vi "Process-Event.vi"(8 "error in":errorcluster, 11 "DAQmx":refnum<class "DAQmx.lvclass">) -> (0 "error out":errorcluster, 3 "DAQmx out":refnum<class "DAQmx.lvclass">)   [LabVIEW 2019, in "DAQmx.lvclass"]
uses:
  DAQmx.lvclass
  C:/Program Files (x86)/National Instruments/LabVIEW 2019/vi.lib/JKI/JKI SMO/SMO/SMO.lvclass
  typedefs/DAQmx.States--enum.ctl
  typedefs/DAQmx.Status--enum.ctl
  <vilib>/JKI/JKI SMO/SMO/SMO.lvclass/SMO.ctl
  DAQmx.lvclass/DAQmx.ctl
  <vilib>/JKI/JKI SMO/SMO/Private/ReftoDVR--SMO.vi
  <vilib>/JKI/JKI SMO/SMO/Protected/Register Process.vi
  <vilib>/JKI/JKI SMO/SMO/SMO.lvclass
panel:
  out "Current State":string
  out "Status":T1
  out "State":T2
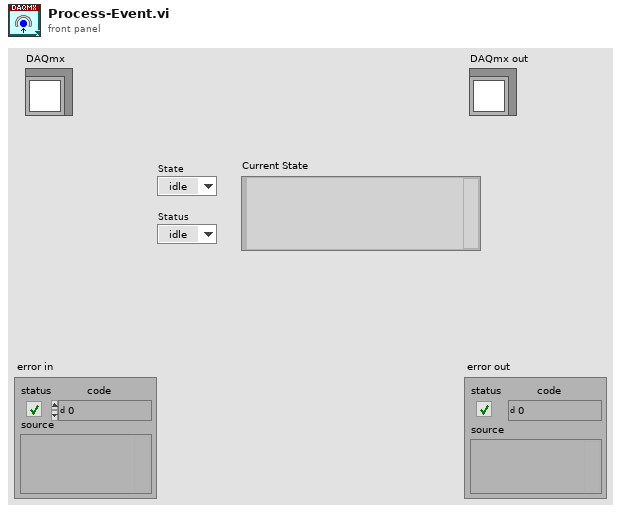
[diagram p1: front panel]
types:
  T1 = typedef "DAQmx.lvclass/DAQmx.Status--enum.ctl" = enum16{"idle", "calibrating", "configuring", "creating", "created", "starting", "started", "stopping", "stopped", "clearing"}
  T2 = typedef "DAQmx.lvclass/DAQmx.States--enum.ctl" = enum16{"idle", "start", "stop", "calibrate", "auto", "exit"}
  T3 = enum32{"Invalid", "Standard", "Closed", "Hidden", "Minimized", "Maximized"}
  T4 = typedef "SMO.lvclass/Protected Events.ctl" = cluster{"StopProcesses":refnum<user-event>, "AbortProcesses":refnum<user-event>, "Config Changed":refnum<user-event>, "Dependency":refnum<user-event>}
  T5 = typedef "DAQmx.lvclass/PrivateEvents--Cluster.ctl" = cluster{"State":refnum<user-event>, "AOconfig":refnum<user-event>, "AIconfig":refnum<user-event>, "Timing":refnum<user-event>}
  T6 = typedef "DAQmx.lvclass/DAQ.Config.AO--Cluster--Array.ctl" = T7[]
  T7 = typedef "DAQmx.lvclass/DAQ.Config.AO--Cluster.ctl" = cluster{"Channels":tag, "Range":T8, "output terminal configuration":i32, "Type":T9}
  T8 = typedef "DAQmx.lvclass/DAQ.Config.AO.Range--enum.ctl" = enum16{"±0.1", "±1.0", "±10.0", ""}
  T9 = typedef "DAQmx.lvclass/DAQ.Config.Device Type--enum.ctl" = enum16{"None", "USB-4431", "PXI-446x"}
  T10 = typedef "DAQmx.lvclass/DAQ.Config.AI--Cluster--Array.ctl" = T11[]
  T11 = typedef "DAQmx.lvclass/DAQ.Config.AI--Cluster.ctl" = cluster{"Channels":tag, "Coupling":T12, "Range":T13, "input terminal configuration":i32, "Type":T9}
  T12 = typedef "DAQmx.lvclass/DAQ.Config.AI.Coupling--enum.ctl" = u16
  T13 = typedef "DAQmx.lvclass/DAQ.Config.AI.Range--enum.ctl" = enum16{"±0.316", "±1.00", "±3.16", "±10.0", "±31.6", "±42.4", ""}
  T14 = typedef "DAQmx.lvclass/DAQ.Config.Timing.Sampling--Cluster.ctl" = cluster{"Fs":dbl, "#s":i32}
  T15 = typedef "DAQmx.lvclass/DeviceInfo--Cluster.ctl" = cluster{"DeviceName":string, "DevIsSimulated":bool, "DeviceSerialNumber":u32, "ProductType":string, "ProductCategory":i32, "ProductNumber":u32, "ChassisNumber":u32, "SlotNumber":u32, "ChassisName":string, "ChassisSerialNumber":u32}
  T16 = typedef "DAQmx.lvclass/DAQ.Calibration--Cluster.ctl" = cluster{"Active Device":string, "SelfCal.LastDate/Time":dbl, "SelfCal.LastTemp":dbl, "DevTemp":dbl, "calibration due?":bool}
  T17 = typedef "DAQmx.lvclass/DAQ.Calibration--Cluster--Array.ctl" = T16[]
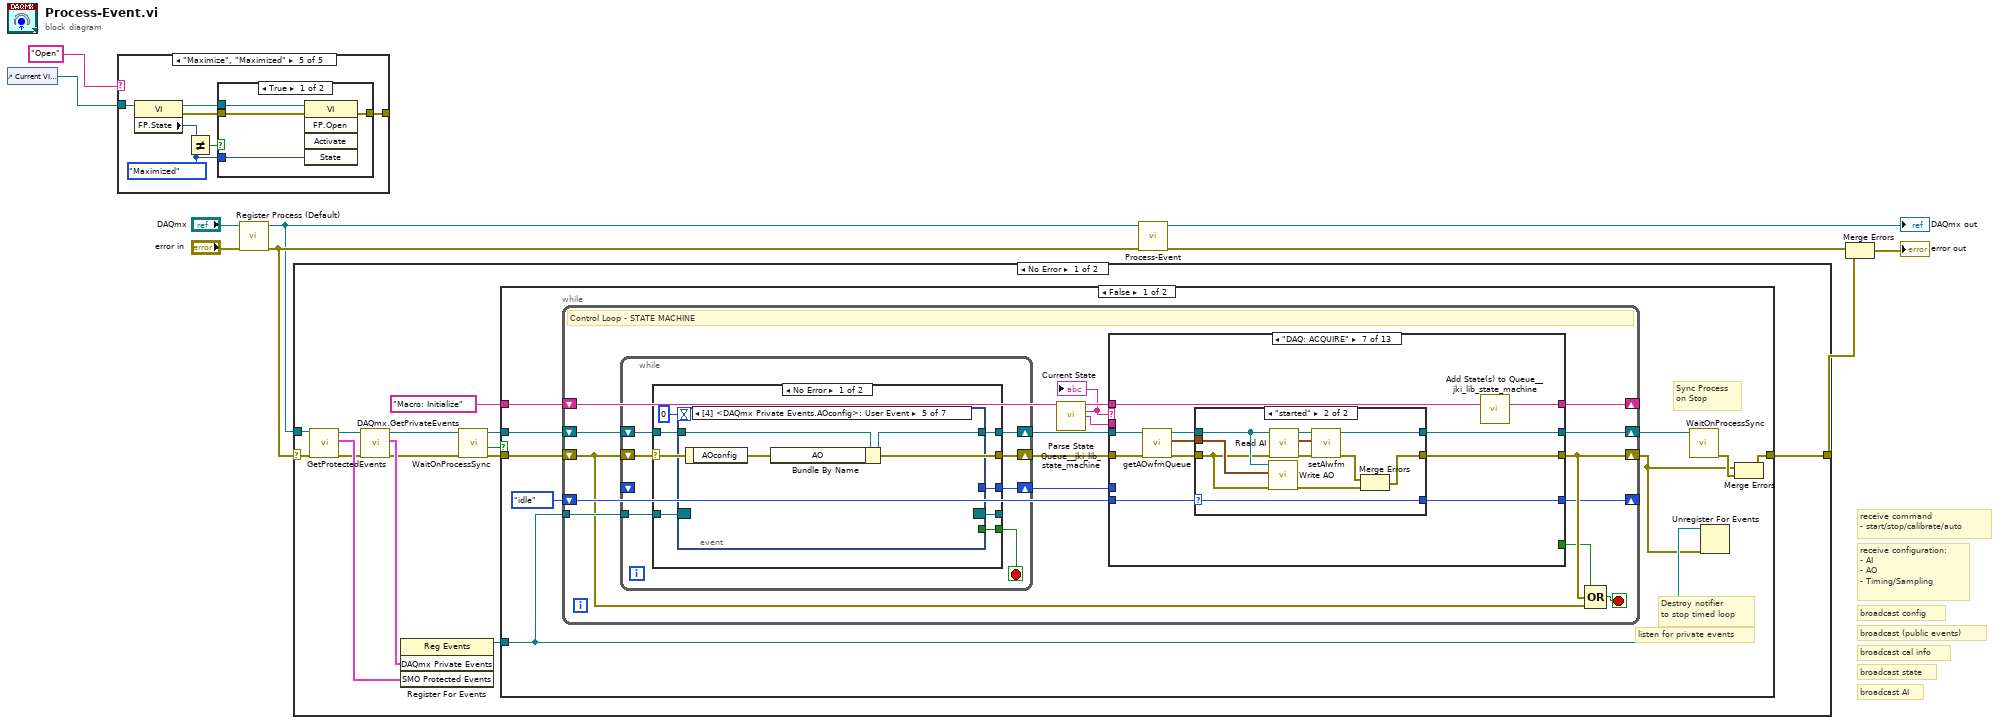
[diagram p0: block diagram]
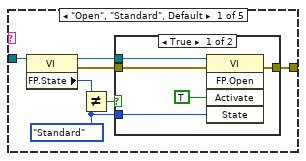
[diagram p2: hidden frame]
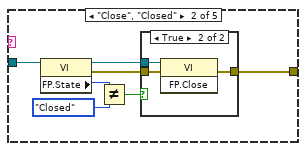
[diagram p4: hidden frame]
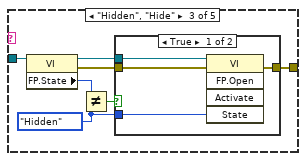
[diagram p6: hidden frame]
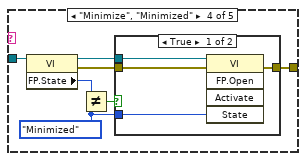
[diagram p8: hidden frame]
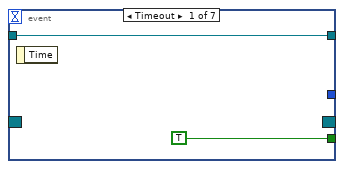
[diagram p11: hidden frame]
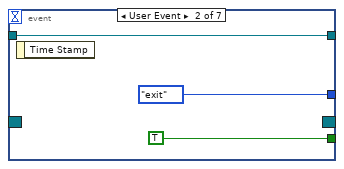
[diagram p12: hidden frame]
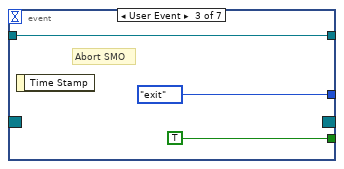
[diagram p13: hidden frame]
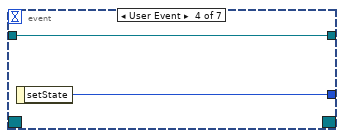
[diagram p14: hidden frame]
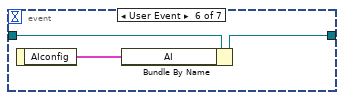
[diagram p15: hidden frame]
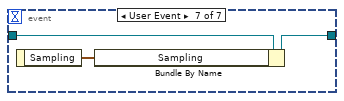
[diagram p16: hidden frame]
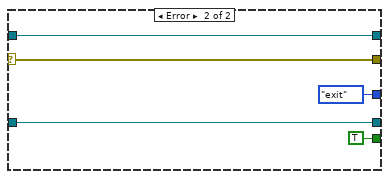
[diagram p17: hidden frame]
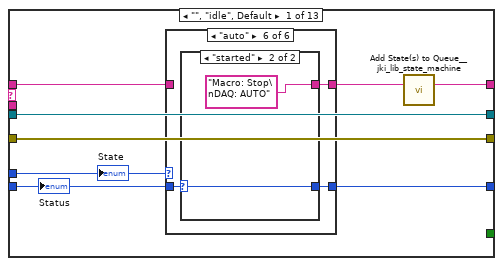
[diagram p18: hidden frame]
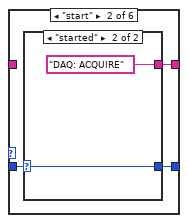
[diagram p20: hidden frame]
diagram:
  # "broadcast (public events)"
  # "receive configuration:\n- AI\n- AO\n- Timing/Sampling"
  # "receive command\n- start/stop/calibrate/auto"
  # "broadcast AI"
  # "broadcast state"
  # "broadcast cal info"
  # "broadcast config"
  n1 = control-ref of="Current VI Reference"() -> (w2:refnum<vi>)
  n2 = case shown="\"Maximize\", \"Maximized\"" "Open" {
    tunnel: [w17 w30 w41 w53 w65] -> _
    tunnel: w2 -> [w16 w28 w40 w52 w64]
    frame "Open", "Standard", Default {
      w11 = T3."Standard" ("State")
      n3 = property class="VI"(reference=w16) -> (reference out=w14:refnum<vi>, error out=w15:errorcluster, "FP.State"=w13:T3)  [unwired: 1 in]
      n4 = Not Equal?(x=w13, y=w11) -> (x != y?=w12:bool)
      n5 = case shown="True" w12 {
        tunnel: [w21 w23] -> w17
        tunnel: w15 -> [w20 w23]
        tunnel: w14 -> [w19 _]
        tunnel: w11 -> [w18 _]
        frame True {
          n6 = invoke class="VI" method="FP.Open"(reference=w19, error in=w20, "Activate"=TRUE, "State"=w18) -> (error out=w21:errorcluster)  [unwired: 1 in, 4 out]
        }
        frame False {
        }
      }
    }
    frame "Close", "Closed" {
      n7 = property class="VI"(reference=w28) -> (reference out=w27:refnum<vi>, error out=w29:errorcluster, "FP.State"=w25:T3)  [unwired: 1 in]
      n8 = Not Equal?(x=w25, y=T3."Closed" ("Front Panel Window:State")) -> (x != y?=w24:bool)
      n9 = case shown="True" w24 {
        tunnel: [w31 w34] -> w30
        tunnel: w29 -> [w31 w33]
        tunnel: w27 -> [_ w32]
        frame False {
        }
        frame True {
          n10 = invoke class="VI" method="FP.Close"(reference=w32, error in=w33) -> (error out=w34:errorcluster)  [unwired: 1 in, 2 out]
        }
      }
    }
    frame "Hidden", "Hide" {
      w35 = T3."Hidden" ("State")
      n11 = property class="VI"(reference=w40) -> (reference out=w38:refnum<vi>, error out=w39:errorcluster, "FP.State"=w37:T3)  [unwired: 1 in]
      n12 = Not Equal?(x=w37, y=w35) -> (x != y?=w36:bool)
      n13 = case shown="True" w36 {
        tunnel: [w45 w46] -> w41
        tunnel: w39 -> [w44 w46]
        tunnel: w38 -> [w43 _]
        tunnel: w35 -> [w42 _]
        frame True {
          n14 = invoke class="VI" method="FP.Open"(reference=w43, error in=w44, "State"=w42) -> (error out=w45:errorcluster)  [unwired: 2 in, 4 out]
        }
        frame False {
        }
      }
    }
    frame "Minimize", "Minimized" {
      w47 = T3."Minimized" ("State")
      n15 = property class="VI"(reference=w52) -> (reference out=w50:refnum<vi>, error out=w51:errorcluster, "FP.State"=w49:T3)  [unwired: 1 in]
      n16 = Not Equal?(x=w49, y=w47) -> (x != y?=w48:bool)
      n17 = case shown="True" w48 {
        tunnel: [w57 w58] -> w53
        tunnel: w51 -> [w56 w58]
        tunnel: w50 -> [w55 _]
        tunnel: w47 -> [w54 _]
        frame True {
          n18 = invoke class="VI" method="FP.Open"(reference=w55, error in=w56, "State"=w54) -> (error out=w57:errorcluster)  [unwired: 2 in, 4 out]
        }
        frame False {
        }
      }
    }
    frame "Maximize", "Maximized" {
      w59 = T3."Maximized" ("State")
      n19 = property class="VI"(reference=w64) -> (reference out=w62:refnum<vi>, error out=w63:errorcluster, "FP.State"=w61:T3)  [unwired: 1 in]
      n20 = Not Equal?(x=w61, y=w59) -> (x != y?=w60:bool)
      n21 = case shown="True" w60 {
        tunnel: [w69 w70] -> w65
        tunnel: w63 -> [w68 w70]
        tunnel: w62 -> [w67 _]
        tunnel: w59 -> [w66 _]
        frame True {
          n22 = invoke class="VI" method="FP.Open"(reference=w67, error in=w68, "State"=w66) -> (error out=w69:errorcluster)  [unwired: 2 in, 4 out]
        }
        frame False {
        }
      }
    }
  }
  n23 = call <vilib>:"Register Process (Default).vi"("error in (no error)"="error in", "SMO"="DAQmx") -> ("error out"=w5:errorcluster, "SelfRef"=w3:refnum<class "DAQmx.lvclass">)  [unwired: 8 in]
  n24 = case shown="No Error" w5 {
    selector: w5 -> [w82 w359]
    tunnel: w3 -> [w83 _]
    tunnel: [w78 w359] -> w10
    frame No Error {
      n25 = call <vilib>:"GetProtectedEvents.vi"("error in (no error)"=w82, "SMO"=w83) -> ("error out"=w76:errorcluster, "SMO Protected Events"=w84:T4, "SMO out"=w75:refnum<class "DAQmx.lvclass">)  [unwired: 7 in]
      n26 = call "DAQmx.GetPrivateEvents.vi"("error in (no error)"=w76, "DAQmx"=w75) -> ("error out"=w71:errorcluster, "DAQmx Private Events"=w74:T5, "DAQmx out"=w72:refnum<class "DAQmx.lvclass">)  [unwired: 7 in]
      n27 = register-events(w74, w84) -> (reference out=w77:refnum<event-registration>)  [unwired: 2 in, 1 out]
      n28 = call <vilib>:"WaitOnProcessSync.vi"("error in (no error)"=w71, "SMO"=w72) -> ("error out"=w80:errorcluster, "Don't run?"=w79:bool, "SMO out"=w81:refnum<class "DAQmx.lvclass">)  [unwired: 7 in]
      n29 = case shown="False" w79 {
        tunnel: w80 -> [w92 w358]
        tunnel: w81 -> [w87 _]
        tunnel: w77 -> [w86 _]
        tunnel: [w90 w358] -> w78
        tunnel: "Macro: Initialize" ("States Out") -> [w88 _]
        frame False {
          # "listen for private events"
          # "Destroy notifier\nto stop timed loop"
          # "Sync Process\non Stop"
          n30 = while {
            shift-right: [w107] -> w93
            shift-left: w87 -> [w102]
            shift-right: [w108] -> w85
            shift-left: w92 -> [w96]
            shift-right: [w106] -> _
            shift-left: w88 -> [w95]
            shift-right: [w105] -> _
            shift-left: DAQmx.Status--enum."idle" ("Status") -> [w97]
            tunnel: w86 -> [w98]
            stop <- w110 stop-if-true
            # "Control Loop - STATE MACHINE"
            n31 = while {
              tunnel: w98 -> [w113]
              shift-right: [w115] -> w100
              shift-left: w102 -> [w117]
              shift-right: [w114] -> w99
              shift-left: w96 -> [w112]
              shift-right: [w116] -> w101
              shift-left: _ -> [_]
              stop <- w111 stop-if-true
              n32 = case shown="No Error" w112 {
                selector: w112 -> [w118 w149]
                tunnel: [w124 w147] -> _
                tunnel: [w123 TRUE] -> w111
                tunnel: [w122 w148] -> w115
                tunnel: w117 -> [w121 w148]
                tunnel: [w120 DAQmx.States--enum."exit" ("setState")] -> w116
                tunnel: w113 -> [w119 w147]
                tunnel: [w118 w149] -> w114
                frame No Error {
                  n33 = event shown="[4] <DAQmx Private Events.AOconfig>: User Event" {
                    selector: w119 -> [_ _ _ _ _ _ _]
                    dyn-events: [_ _ _ _ _ _ _] -> w124
                    timeout: 0 -> [_ _ _ _ _ _ _]
                    tunnel: [TRUE TRUE TRUE _ _ _ _] -> w123
                    tunnel: [w127 w129 w132 w135 w137 w141 w143] -> w122
                    tunnel: w121 -> [w127 w129 w132 w135 w136 w140 w142]
                    tunnel: [_ DAQmx.States--enum."exit" ("setState") DAQmx.States--enum."exit" ("setState") w134 _ _ _] -> w120
                    event Timeout {
                      n34 = event-data() -> ()  [unwired: 1 in, 1 out]
                    }
                    event User Event {
                      n35 = event-data() -> ()  [unwired: 1 in, 1 out]
                    }
                    event User Event {
                      # "Abort SMO"
                      n36 = event-data() -> ()  [unwired: 1 in, 1 out]
                    }
                    event User Event {
                      n37 = event-data() -> ("setState"=w134:T2)  [unwired: 1 in]
                    }
                    event User Event {
                      n38 = event-data() -> ("AOconfig"=w138:T6)  [unwired: 1 in]
                      n39 = Bundle By Name(cluster=w136, "AO"=w138) -> (w137:refnum<class "DAQmx.lvclass">)
                    }
                    event User Event {
                      n40 = event-data() -> ("AIconfig"=w139:T10)  [unwired: 1 in]
                      n41 = Bundle By Name(cluster=w140, "AI"=w139) -> (w141:refnum<class "DAQmx.lvclass">)
                    }
                    event User Event {
                      n42 = event-data() -> ("Sampling"=w144:T14)  [unwired: 1 in]
                      n43 = Bundle By Name(cluster=w142, "Sampling"=w144) -> (w143:refnum<class "DAQmx.lvclass">)
                    }
                  }
                }
                frame Error {
                }
              }
            }
            n44 = call <vilib>:"Parse State Queue__jki_lib_state_machine.vi"("State Queue"=w95) -> ("Remaining States"=w109:string, "Current State"=w103:string, "Arguments"=w104:string)  [unwired: 12 in]
            "Current State" <- w103
            n45 = case shown="\"DAQ: ACQUIRE\"" w103 {
              tunnel: w100 -> [w157 w206 w222 w240 w265 w273 w288 w313 w325 w335 w338 w344 w351]
              tunnel: [w157 w195 w216 w231 w259 w276 w291 w311 w322 w335 w338 w344 w352] -> w107
              tunnel: [w156 w196 w215 w232 w260 w277 w294 w312 w321 w334 w339 w345 w350] -> w108
              tunnel: w99 -> [w156 w204 w221 w239 w266 w272 w287 w314 w330 w334 w339 w345 w349]
              tunnel: w104 -> [_ _ _ w246 _ _ _ _ _ _ _ _ _]
              tunnel: w109 -> [w150 w208 w230 w245 w267 w282 w293 w319 w331 _ w341 w347 w356]
              tunnel: [w155 w209 w229 w244 w268 w283 w292 w320 w332 "DAQ: Query Hardware" ("States Out") w342 w348 w357] -> w106
              tunnel: [w152 w197 w220 w234 w257 w274 w289 w309 w323 w333 w337 w343 w354] -> w105
              tunnel: w97 -> [w153 _ _ _ _ _ w290 _ _ w333 w337 w343 w354]
              tunnel: w101 -> [w154 _ _ _ _ _ _ _ _ _ _ _ _]
              tunnel: [_ _ _ _ _ _ _ _ _ _ _ _ TRUE] -> w94
              frame "", "idle", Default {
                n46 = case shown="\"auto\"" w154 {
                  tunnel: w153 -> [w158 w162 w169 w176 w183 w190]
                  tunnel: [w159 w161 w168 w175 w182 w189] -> w151
                  tunnel: [w158 w160 w167 w174 w181 w188] -> w152
                  tunnel: w150 -> [w159 _ _ _ _ _]
                  frame "idle", Default {
                  }
                  frame "start" {
                    n47 = case shown="\"started\"" w162 {
                      selector: w162 -> [w163 w165]
                      tunnel: ["Macro: Start" ("State(s) in (\"\")") "DAQ: ACQUIRE" ("State(s) in (\"\")")] -> w161
                      tunnel: [w163 w165] -> w160
                      frame Default {
                      }
                      frame "started" {
                      }
                    }
                  }
                  frame "stop" {
                    n48 = case shown="Default" w169 {
                      selector: w169 -> [w170 w172]
                      tunnel: ["" ("State(s) in (\"\")") "Macro: Stop" ("State(s) in (\"\")")] -> w168
                      tunnel: [w170 w172] -> w167
                      frame Default {
                      }
                      frame "started" {
                      }
                    }
                  }
                  frame "exit" {
                    n49 = case shown="\"started\"" w176 {
                      selector: w176 -> [w177 w179]
                      tunnel: ["exit" ("State(s) in (\"\")") "Macro: Stop\nexit" ("State(s) in (\"\")")] -> w175
                      tunnel: [w177 w179] -> w174
                      frame Default {
                      }
                      frame "started" {
                      }
                    }
                  }
                  frame "calibrate" {
                    n50 = case shown="Default" w183 {
                      selector: w183 -> [w184 w186]
                      tunnel: ["DAQ: CALIBRATE" ("State(s) in (\"\")") "Macro: Stop\nDAQ: CALIBRATE" ("State(s) in (\"\")")] -> w182
                      tunnel: [w184 w186] -> w181
                      frame Default {
                      }
                      frame "started" {
                      }
                    }
                  }
                  frame "auto" {
                    n51 = case shown="\"started\"" w190 {
                      selector: w190 -> [w191 w193]
                      tunnel: ["DAQ: AUTO" ("State(s) in (\"\")") "Macro: Stop\nDAQ: AUTO" ("State(s) in (\"\")")] -> w189
                      tunnel: [w191 w193] -> w188
                      frame Default {
                      }
                      frame "started" {
                      }
                    }
                  }
                }
                n52 = call <vilib>:"Add State(s) to Queue__jki_lib_state_machine.vi"("State(s) in (\"\")"=w151) -> ("States Out"=w155:string)  [unwired: 14 in]
                "State" <- w154
                "Status" <- w153
              }
              frame "DAQ: Query Hardware" {
                w197 = DAQmx.Status--enum."idle" ("setStatus")
                n53 = call "setStatus.vi"("error in (no error)"=w204, "Status"=DAQmx.Status--enum."configuring" ("setStatus"), "DAQmx in"=w206) -> ("error out"=w205:errorcluster, "DAQmx out"=w207:refnum<class "DAQmx.lvclass">)  [unwired: 7 in]
                n54 = call "Enumerate And Sort Devices.vi"("error in (no error)"=w205, "DAQmx in"=w207) -> ("error out"=w201:errorcluster, "Devices (sorted)"=w203:T15[], "DAQmx out"=w202:refnum<class "DAQmx.lvclass">)  [unwired: 7 in]
                n55 = call "setDevices.vi"("error in (no error)"=w201, "Devices"=w203, "DAQmx in"=w202) -> ("error out"=w199:errorcluster, "DAQmx out"=w200:refnum<class "DAQmx.lvclass">)  [unwired: 7 in]
                n56 = call "setStatus.vi"("error in (no error)"=w199, "Status"=w197, "DAQmx in"=w200) -> ("error out"=w196:errorcluster, "DAQmx out"=w195:refnum<class "DAQmx.lvclass">)  [unwired: 7 in]
                n57 = call <vilib>:"Add State(s) to Queue__jki_lib_state_machine.vi"("State(s) in (\"\")"=w208) -> ("States Out"=w209:string)  [unwired: 14 in]
              }
              frame "DAQ: AUTO" {
                w220 = DAQmx.Status--enum."idle" ("setStatus")
                n58 = call "setStatus.vi"("error in (no error)"=w221, "Status"=DAQmx.Status--enum."configuring" ("setStatus"), "DAQmx in"=w222) -> ("error out"=w224:errorcluster, "DAQmx out"=w223:refnum<class "DAQmx.lvclass">)  [unwired: 7 in]
                n59 = call "Auto Configure DAQ.vi"("error in (no error)"=w224, "DAQmx in"=w223) -> ("error out"=w228:errorcluster, "Configuration.AO"=w218:T6, "Configuration.AI"=w210:T10, "DAQmx out"=w227:refnum<class "DAQmx.lvclass">, "Devices"=w226:T15[])  [unwired: 5 in]
                n60 = call "setDevices.vi"("error in (no error)"=w228, "Devices"=w226, "DAQmx in"=w227) -> ("error out"=w225:errorcluster, "DAQmx out"=w217:refnum<class "DAQmx.lvclass">)  [unwired: 7 in]
                n61 = call "setAIconfig(private).vi"("error in (no error)"=w225, "AIconfig"=w210, "DAQmx in"=w217) -> ("error out"=w213:errorcluster, "DAQmx out"=w214:refnum<class "DAQmx.lvclass">)  [unwired: 7 in]
                n62 = call "setAOconfig(private).vi"("error in (no error)"=w213, "AOconfig"=w218, "DAQmx in"=w214) -> ("error out"=w211:errorcluster, "DAQmx out"=w212:refnum<class "DAQmx.lvclass">)  [unwired: 7 in]
                n63 = call <vilib>:"Add State(s) to Queue__jki_lib_state_machine.vi"("State(s) in (\"\")"=w230) -> ("States Out"=w229:string)  [unwired: 14 in]
                n64 = call "setStatus.vi"("error in (no error)"=w211, "Status"=w220, "DAQmx in"=w212) -> ("error out"=w215:errorcluster, "DAQmx out"=w216:refnum<class "DAQmx.lvclass">)  [unwired: 7 in]
              }
              frame "DAQ: CALIBRATE" {
                w234 = DAQmx.Status--enum."idle" ("Status")
                n65 = call "setStatus.vi"("error in (no error)"=w239, "Status"=DAQmx.Status--enum."calibrating" ("setStatus"), "DAQmx in"=w240) -> ("error out"=w237:errorcluster, "DAQmx out"=w236:refnum<class "DAQmx.lvclass">)  [unwired: 7 in]
                n66 = case shown="\"Check\", Default" w246 {
                  tunnel: w236 -> [w251 w256]
                  tunnel: [w250 w255] -> w242
                  tunnel: [w248 w254] -> w243
                  tunnel: w237 -> [w249 w253]
                  tunnel: [w247 w252] -> w241
                  frame "Calibrate" {
                    n67 = call "Calibrate.vi"("error in (no error)"=w249, "DAQmx in"=w251) -> ("error out"=w248:errorcluster, "Cal Info"=w247:T16[], "DAQmx out"=w250:refnum<class "DAQmx.lvclass">)  [unwired: 7 in]
                  }
                  frame "Check", Default {
                    n68 = call "Get Calibration.vi"("error in (no error)"=w253, "DAQmx in"=w256) -> ("error out"=w254:errorcluster, "Calibration"=w252:T17, "DAQmx out"=w255:refnum<class "DAQmx.lvclass">)  [unwired: 7 in]
                  }
                }
                n69 = call "setCalibration.vi"("error in (no error)"=w243, "Calibration"=w241, "DAQmx in"=w242) -> ("error out"=w233:errorcluster, "DAQmx out"=w235:refnum<class "DAQmx.lvclass">)  [unwired: 7 in]
                n70 = call "setStatus.vi"("error in (no error)"=w233, "Status"=w234, "DAQmx in"=w235) -> ("error out"=w232:errorcluster, "DAQmx out"=w231:refnum<class "DAQmx.lvclass">)  [unwired: 7 in]
                n71 = call <vilib>:"Add State(s) to Queue__jki_lib_state_machine.vi"("State(s) in (\"\")"=w245) -> ("States Out"=w244:string)  [unwired: 14 in]
              }
              frame "DAQ: CREATE" {
                w257 = DAQmx.Status--enum."created" ("Status")
                n72 = call "setStatus.vi"("error in (no error)"=w266, "Status"=DAQmx.Status--enum."creating", "DAQmx in"=w265) -> ("error out"=w263:errorcluster, "DAQmx out"=w264:refnum<class "DAQmx.lvclass">)  [unwired: 7 in]
                n73 = call "Create Acquisition.vi"("error in"=w263, "DAQmx in"=w264) -> ("error out"=w261:errorcluster, "DAQmx out"=w262:refnum<class "DAQmx.lvclass">)  [unwired: 8 in]
                n74 = call "setStatus.vi"("error in (no error)"=w261, "Status"=w257, "DAQmx in"=w262) -> ("error out"=w260:errorcluster, "DAQmx out"=w259:refnum<class "DAQmx.lvclass">)  [unwired: 7 in]
                n75 = call <vilib>:"Add State(s) to Queue__jki_lib_state_machine.vi"("State(s) in (\"\")"=w267) -> ("States Out"=w268:string)  [unwired: 14 in]
              }
              frame "DAQ: START" {
                w274 = DAQmx.Status--enum."started" ("Status")
                n76 = call "getAOwfmQueue.vi"("error in (no error)"=w272, "DAQmx in"=w273) -> ("error out"=w270:errorcluster, "AOwfm"=w269:waveform(dbl)[], "DAQmx out"=w271:refnum<class "DAQmx.lvclass">)  [unwired: 6 in, 1 out]
                n77 = call "setStatus.vi"("error in (no error)"=w270, "Status"=DAQmx.Status--enum."starting", "DAQmx in"=w271) -> ("error out"=w280:errorcluster, "DAQmx out"=w281:refnum<class "DAQmx.lvclass">)  [unwired: 7 in]
                n78 = call "Start Acquisition.vi"("error in"=w280, "WFM in"=w269, "DAQmx in"=w281) -> ("error out"=w278:errorcluster, "DAQmx out"=w279:refnum<class "DAQmx.lvclass">)  [unwired: 7 in]
                n79 = call "setStatus.vi"("error in (no error)"=w278, "Status"=w274, "DAQmx in"=w279) -> ("error out"=w277:errorcluster, "DAQmx out"=w276:refnum<class "DAQmx.lvclass">)  [unwired: 7 in]
                n80 = call <vilib>:"Add State(s) to Queue__jki_lib_state_machine.vi"("State(s) in (\"\")"=w282) -> ("States Out"=w283:string)  [unwired: 14 in]
              }
              frame "DAQ: ACQUIRE" {
                n81 = call "getAOwfmQueue.vi"("error in (no error)"=w287, "DAQmx in"=w288) -> ("error out"=w286:errorcluster, "AOwfm"=w284:waveform(dbl)[], "DAQmx out"=w285:refnum<class "DAQmx.lvclass">)  [unwired: 6 in, 1 out]
                n82 = case shown="\"started\"" w290 {
                  selector: w290 -> [w295 w300]
                  tunnel: [w296 w307] -> w294
                  tunnel: w286 -> [w296 w298]
                  tunnel: [w297 w303] -> w291
                  tunnel: w285 -> [w297 w301]
                  tunnel: w284 -> [_ w299]
                  tunnel: [w295 w300] -> w289
                  frame Default {
                  }
                  frame "started" {
                    n83 = call "Write AO.vi"("error in (no error)"=w298, "AO []"=w299, "DAQmx in"=w301) -> ("error out"=w308:errorcluster)  [unwired: 5 in, 3 out]
                    n84 = call "Read AI.vi"("error in"=w298, "DAQmx in"=w301) -> ("error out"=w304:errorcluster, "AI []"=w306:waveform(dbl)[], "DAQmx out"=w305:refnum<class "DAQmx.lvclass">)  [unwired: 6 in, 1 out]
                    n85 = call "setAIwfm.vi"("error in (no error)"=w304, "AIwfm"=w306, "DAQmx in"=w305) -> ("error out"=w302:errorcluster, "DAQmx out"=w303:refnum<class "DAQmx.lvclass">)  [unwired: 7 in]
                    n86 = Merge Errors(w302, w308) -> (w307:errorcluster)
                  }
                }
                n87 = call <vilib>:"Add State(s) to Queue__jki_lib_state_machine.vi"("State(s) in (\"\")"=w293) -> ("States Out"=w292:string)  [unwired: 14 in]
              }
              frame "DAQ: STOP" {
                w309 = DAQmx.Status--enum."stopped" ("Status")
                n88 = call "setStatus.vi"("error in (no error)"=w314, "Status"=DAQmx.Status--enum."stopping", "DAQmx in"=w313) -> ("error out"=w317:errorcluster, "DAQmx out"=w318:refnum<class "DAQmx.lvclass">)  [unwired: 7 in]
                n89 = call "Stop Acquisition.vi"("error in (no error)"=w317, "DAQmx in"=w318) -> ("error out"=w315:errorcluster, "DAQmx out"=w316:refnum<class "DAQmx.lvclass">)  [unwired: 8 in]
                n90 = call "setStatus.vi"("error in (no error)"=w315, "Status"=w309, "DAQmx in"=w316) -> ("error out"=w312:errorcluster, "DAQmx out"=w311:refnum<class "DAQmx.lvclass">)  [unwired: 7 in]
                n91 = call <vilib>:"Add State(s) to Queue__jki_lib_state_machine.vi"("State(s) in (\"\")"=w319) -> ("States Out"=w320:string)  [unwired: 14 in]
              }
              frame "DAQ: CLEAR" {
                w323 = DAQmx.Status--enum."idle" ("Status")
                n92 = call "setStatus.vi"("error in (no error)"=w330, "Status"=DAQmx.Status--enum."clearing", "DAQmx in"=w325) -> ("error out"=w328:errorcluster, "DAQmx out"=w329:refnum<class "DAQmx.lvclass">)  [unwired: 7 in]
                n93 = call "Clear.vi"("error in (no error)"=w328, "DAQmx in"=w329) -> ("error out"=w326:errorcluster, "DAQmx out"=w327:refnum<class "DAQmx.lvclass">)  [unwired: 8 in]
                n94 = call "setStatus.vi"("error in (no error)"=w326, "Status"=w323, "DAQmx in"=w327) -> ("error out"=w321:errorcluster, "DAQmx out"=w322:refnum<class "DAQmx.lvclass">)  [unwired: 7 in]
                n95 = call <vilib>:"Add State(s) to Queue__jki_lib_state_machine.vi"("State(s) in (\"\")"=w331) -> ("States Out"=w332:string)  [unwired: 14 in]
              }
              frame "Macro: Initialize" {
              }
              frame "Macro: Start" {
                n96 = call <vilib>:"Add State(s) to Queue__jki_lib_state_machine.vi"("State(s) in Front (\"\")"="DAQ: CREATE\nDAQ: START\nDAQ: ACQUIRE" ("State(s) in Front (\"\")"), "State(s) in (\"\")"=w341) -> ("States Out"=w342:string)  [unwired: 13 in]
              }
              frame "Macro: Stop" {
                n97 = call <vilib>:"Add State(s) to Queue__jki_lib_state_machine.vi"("State(s) in Front (\"\")"="DAQ: STOP\nDAQ: CLEAR" ("State(s) in Front (\"\")"), "State(s) in (\"\")"=w347) -> ("States Out"=w348:string)  [unwired: 13 in]
              }
              frame "exit" {
                n98 = call <vilib>:"SelfTerminate.vi"("error in (no error)"=w349, "SMO in"=w351) -> ("error out"=w350:errorcluster, "SMO out"=w352:refnum<class "DAQmx.lvclass">)  [unwired: 8 in]
                n99 = call <vilib>:"Add State(s) to Queue__jki_lib_state_machine.vi"("State(s) in Front (\"\")"="" ("State(s) in Front (\"\")"), "State(s) in (\"\")"=w356) -> ("States Out"=w357:string)  [unwired: 13 in]
              }
            }
            n100 = Compound Arithmetic op=OR(w94, w108, w96) -> (w110:bool)
          }
          n101 = call <vilib>:"WaitOnProcessSync.vi"("SMO"=w93) -> ("error out"=w91:errorcluster)  [unwired: 8 in, 2 out]
          n102 = Unregister For Events(event registration refnum=w86, error in=w85) -> ()  [unwired: 1 out]
          n103 = Merge Errors(w85, w91) -> (w90:errorcluster)
        }
        frame True {
        }
      }
    }
    frame Error {
    }
  }
  n104 = call-parent "Process-Event.vi"("error in"=w5, "SMO"=w3) -> ("error out"=w9:errorcluster, "SMO out"=→"DAQmx out":refnum<class "DAQmx.lvclass">)  [unwired: 8 in]
  n105 = Merge Errors(w9, w10) -> (→"error out":errorcluster)
